vi "Com_SECS Equipment _SECS Packet Unflatten.vi"(8 "error in":errorcluster, 11 "Data":string) -> (0 "error out":errorcluster, 3 "SECS Packet":T1)   [LabVIEW 2016]
uses:
  Data Def/Com_SECS Equipment _SECS Packet.ctl
  Data Def/Com_SECS Equipment _Message Type.ctl
  Data Def/Com_SECS Equipment _Protocol Type.ctl
  Data Def/Com_SECS Equipment _Stream Type.ctl
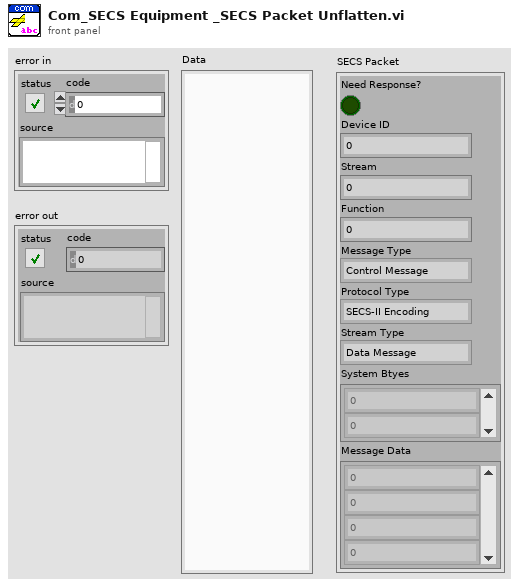
[diagram p1: front panel]
types:
  T1 = typedef "Com_SECS Equipment _SECS Packet.ctl" = cluster{"Need Response?":bool, "Device ID":u16, "Stream":u8, "Function":u8, "Message Type":T2, "Protocol Type":T3, "Stream Type":T4, "System Btyes":u8[], "Message Data":u8[]}
  T2 = typedef "Com_SECS Equipment _Message Type.ctl" = enum16{"Control Message", "Data Message"}
  T3 = typedef "Com_SECS Equipment _Protocol Type.ctl" = enum16{"SECS-II Encoding", "Reserved"}
  T4 = typedef "Com_SECS Equipment _Stream Type.ctl" = enum16{"Data Message", "Select.req", "Select.rsp", "Deselect.req", "Deselect.rsp", "Linktest.req", "Linktest.rsp", "Reject.req", "Separate.req", "Reserve"}
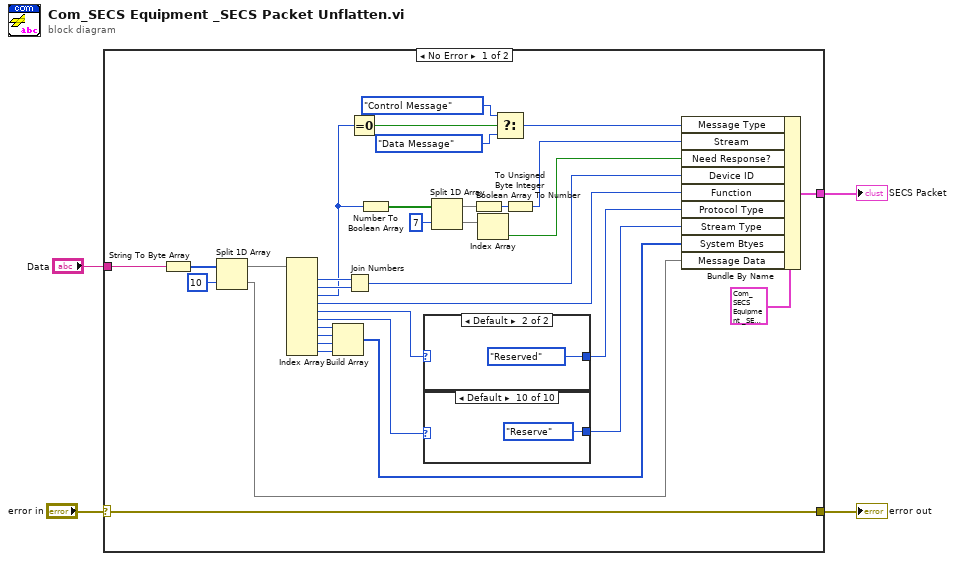
[diagram p0: block diagram]
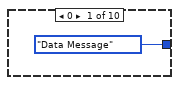
[diagram p2: hidden frame]
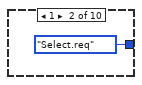
[diagram p3: hidden frame]
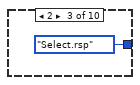
[diagram p4: hidden frame]
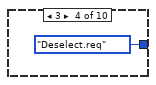
[diagram p5: hidden frame]
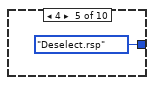
[diagram p6: hidden frame]
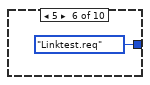
[diagram p7: hidden frame]
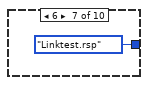
[diagram p8: hidden frame]
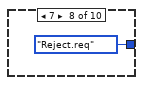
[diagram p9: hidden frame]
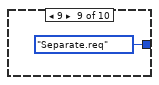
[diagram p10: hidden frame]
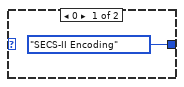
[diagram p11: hidden frame]
diagram:
  n1 = case shown="No Error" "error in" {
    selector: "error in" -> [w23 w50]
    tunnel: [w23 w50] -> w2
    tunnel: "Data" -> [w22 _]
    tunnel: [w15 _] -> w1
    frame No Error {
      n2 = String To Byte Array(string=w22) -> (unsigned byte array=w32:u8[])
      n3 = Split 1D Array(array=w32, index=10) -> (first subarray=w25:u8[], second subarray=w24:u8[])
      n4 = Index Array(array=w25) -> (element #1=w37:u8, element #2=w36:u8, element #3=w17:u8, element #4=w35:u8, element #5=w34:u8, element #6=w33:u8, element #7=w30:u8, element #8=w31:u8, element #9=w28:u8, element #10=w27:u8)  [unwired: 10 in]
      n5 = Build Array(w30, w31, w28, w27) -> (w29:u8[])
      n6 = Join Numbers(hi=w37, lo=w36) -> ((hi.lo)=w18:u16)
      n7 = Equal To 0?(x=w17) -> (x = 0?=w16:bool)
      n8 = Number To Boolean Array(number=w17) -> (Boolean array=w21:bool[])
      n9 = case shown="Default" w34 {
        tunnel: [Com_SECS_Equipment__Protocol_Type."SECS-II Encoding" ("Protocol Type") Com_SECS_Equipment__Protocol_Type."Reserved" ("Protocol Type")] -> w6
        frame 0 {
        }
        frame Default {
        }
      }
      n10 = case shown="Default" w33 {
        tunnel: [Com_SECS_Equipment__Stream_Type."Data Message" ("Stream Type") Com_SECS_Equipment__Stream_Type."Select.req" ("Stream Type") Com_SECS_Equipment__Stream_Type."Select.rsp" ("Stream Type") Com_SECS_Equipment__Stream_Type."Deselect.req" ("Stream Type") Com_SECS_Equipment__Stream_Type."Deselect.rsp" ("Stream Type") Com_SECS_Equipment__Stream_Type."Linktest.req" ("Stream Type") Com_SECS_Equipment__Stream_Type."Linktest.rsp" ("Stream Type") Com_SECS_Equipment__Stream_Type."Reject.req" ("Stream Type") Com_SECS_Equipment__Stream_Type."Separate.req" ("Stream Type") Com_SECS_Equipment__Stream_Type."Reserve" ("Stream Type")] -> w5
        frame 0 {
        }
        frame 1 {
        }
        frame 2 {
        }
        frame 3 {
        }
        frame 4 {
        }
        frame 5 {
        }
        frame 6 {
        }
        frame 7 {
        }
        frame 9 {
        }
        frame Default {
        }
      }
      n11 = Split 1D Array(array=w21, index=7) -> (first subarray=w14:bool[], second subarray=w13:bool[])
      n12 = Boolean Array To Number(Boolean array=w14) -> (number=w19:u32)
      n13 = Index Array(array=w13) -> (element=w7:bool)  [unwired: 1 in]
      n14 = Select(t=Com_SECS_Equipment__Message_Type."Control Message" ("Message Type"), s=w16, f=Com_SECS_Equipment__Message_Type."Data Message" ("Message Type")) -> (s? t:f=w9:T2)
      n15 = To Unsigned Byte Integer(number=w19) -> (unsigned 8bit integer=w8:u8)
      n16 = Bundle By Name(cluster=T1 {"Need Response?"=FALSE, "Device ID"=0, "Stream"=0, "Function"=0, "Message Type"=enum."Control Message", "Protocol Type"=enum."SECS-II Encoding", "Stream Type"=enum."Data Message", "System Btyes"=[], "Message Data"=[]} ("SECS Packet"), "Message Type"=w9, "Stream"=w8, "Need Response?"=w7, "Device ID"=w18, "Function"=w35, "Protocol Type"=w6, "Stream Type"=w5, "System Btyes"=w29, "Message Data"=w24) -> (w15:T1)
    }
    frame Error {
    }
  }
  "error out" <- w2
  "SECS Packet" <- w1
